vi "ForLoop.vi"(8 "error in":errorcluster, 11 "reference":refnum<vi>) -> (0 "error out":errorcluster, 3 "ForLoop out":refnum<class "ForLoop.lvclass">)   [LabVIEW 2014, in "Raspberry Pi Compatible Compiler for LabVIEW.lvlib" / "ForLoop.lvclass"]
uses:
  ForLoop.lvclass
  ForLoop.lvclass/ForLoop.ctl
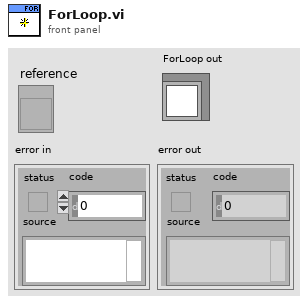
[diagram p1: front panel]
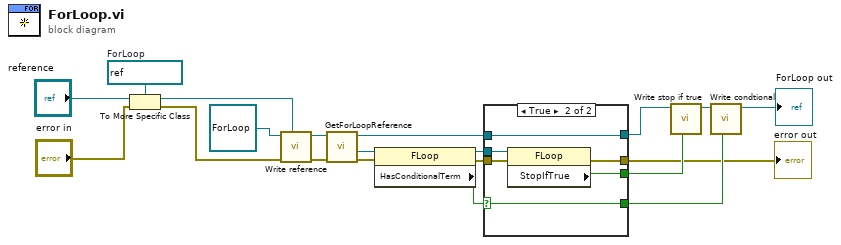
[diagram p0: block diagram]
diagram:
  w19 = refnum<vi> refnum  # ForLoop
  n1 = To More Specific Class(target class=w19, reference="reference", error in="error in") -> (specific class reference=w16:refnum<vi>, error out=w17:errorcluster)
  n2 = call-dynamic "Write reference.vi"("reference"=w16, "error in"=w17, "GObject in"=refnum<class "ForLoop.lvclass"> refnum ("ForLoop in")) -> ("error out"=w14:errorcluster, "GObject out"=w15:refnum<class "ForLoop.lvclass">)  [unwired: 5 in]
  n3 = call "GetForLoopReference.vi"("error in"=w14, "ForLoop in"=w15) -> ("error out"=w9:errorcluster, "reference out"=w13:refnum<vi>, "ForLoop out"=w12:refnum<class "ForLoop.lvclass">)  [unwired: 7 in]
  n4 = property class="FLoop"(reference=w13, error in=w9) -> (reference out=w7:refnum<vi>, error out=w8:errorcluster, "HasConditionalTerm"=w10:bool)
  n5 = case shown="True" w10 {
    selector: w10 -> [w22 w26]
    tunnel: w12 -> [w23 w25]
    tunnel: [w23 w25] -> w6
    tunnel: w8 -> [w21 w28]
    tunnel: w7 -> [_ w29]
    tunnel: [_ w27] -> w5
    tunnel: [w22 w26] -> w2
    tunnel: [w21 w24] -> w1
    frame False {
    }
    frame True {
      n6 = property class="FLoop"(reference=w29, error in=w28) -> (error out=w24:errorcluster, "StopIfTrue"=w27:bool)  [unwired: 1 out]
    }
  }
  "error out" <- w1
  n7 = call "Write stop if true.vi"("stop if true"=w5, "ForLoop in"=w6) -> ("ForLoop out"=w4:refnum<class "ForLoop.lvclass">)  [unwired: 7 in]
  n8 = call "Write condtional.vi"("condtional"=w2, "ForLoop in"=w4) -> ("ForLoop out"=→"ForLoop out":refnum<class "ForLoop.lvclass">)  [unwired: 7 in]
